vi "StopAcquisition.vi"(8 "error in (no error)":errorcluster) -> (0 "error out":errorcluster, 3 "AcquisitionIsStopped":bool)   [LabVIEW 2014]
uses:
  USBAnalyzerEllisysDll/Debug/USBAnalyzerEllisysDll.dll
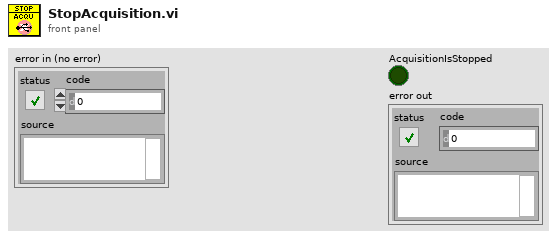
[diagram p1: front panel]
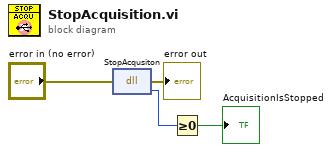
[diagram p0: block diagram]
diagram:
  n1 = dll-call lib="PTH2labs CUsersMichał\tDocumentsEllisysAnalyzerUSBAnalyzerEllisysDllDebugUSBAnalyzerEllisysDll.dll" fn="StopAcqusiton"(error in="error in (no error)") -> (error out=→"error out":errorcluster, "return type"=w4:i32)  [unwired: 2 in, 1 out]
  n2 = Greater Or Equal To 0?(x=w4) -> (x >= 0?=→"AcquisitionIsStopped":bool)
